vi "No Target LED.vi"(11 "Thing 1":bool) -> (3 "Flashy the LED":bool)   [LabVIEW 2011]
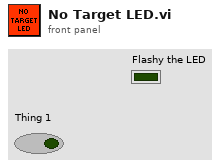
[diagram p1: front panel]
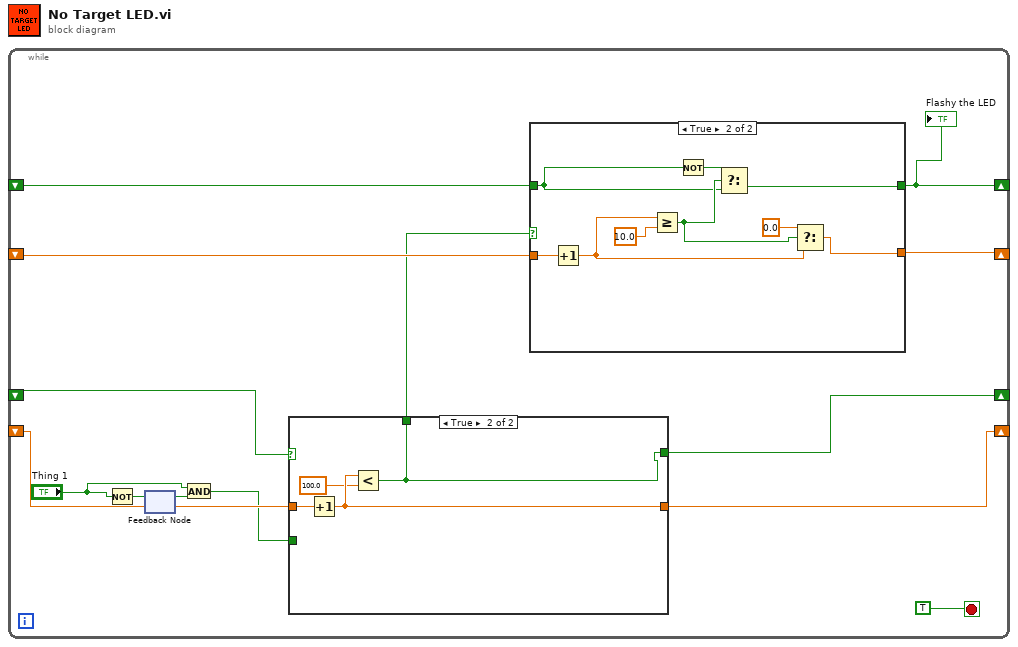
[diagram p0: block diagram]
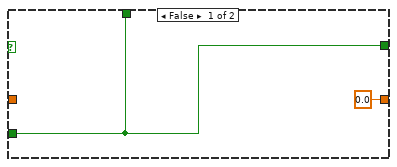
[diagram p2: hidden frame]
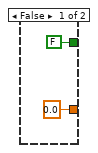
[diagram p3: hidden frame]
diagram:
  n1 = while {
    shift-right: [w13] -> _
    shift-left: _ -> [w14]
    shift-right: [w9] -> _
    shift-left: _ -> [w8]
    shift-right: [w5] -> _
    shift-left: _ -> [w6]
    shift-right: [w2] -> _
    shift-left: _ -> [w7]
    stop <- TRUE stop-if-true
    n2 = Not(x="Thing 1") -> (.not. x?=w12:bool)
    n3 = feedback-in #1(w12) -> ()
    n4 = feedback #1() -> (w11:bool)  [unwired: 1 in]
    n5 = And(x="Thing 1", y=w11) -> (x .and. y?=w1:bool)
    n6 = case shown="True" w8 {
      tunnel: [w15 w17] -> w9
      tunnel: w1 -> [w15 _]
      tunnel: w6 -> [_ w20]
      tunnel: [0.0 w19] -> w5
      tunnel: [w15 w17] -> w4
      frame False {
      }
      frame True {
        n7 = Increment(x=w20) -> (x+1=w19:dbl)
        n8 = Less?(x=w19, y=100.0 ("y 2")) -> (x < y?=w17:bool)
      }
    }
    n9 = case shown="True" w4 {
      tunnel: w14 -> [_ w31]
      tunnel: [0.0 ("t") w30] -> w13
      tunnel: [FALSE ("Latched") w23] -> w2
      tunnel: w7 -> [_ w24]
      frame False {
      }
      frame True {
        n10 = Increment(x=w31) -> (x+1=w27:dbl)
        n11 = Greater Or Equal?(x=w27, y=10.0) -> (x >= y?=w25:bool)
        n12 = Not(x=w24) -> (.not. x?=w26:bool)
        n13 = Select(t=w26, s=w25, f=w24) -> (s? t:f=w23:bool)
        n14 = Select(t=0.0, s=w25, f=w27) -> (s? t:f=w30:dbl)
      }
    }
    "Flashy the LED" <- w2
  }
